vi "InfoGui.vi"(7 "_onebutton(F)":bool caption="one button (F)", 9 "_Arg":variant[](array[variant]), 10 "_Msg":T1) -> (2 "ok":bool)   [LabVIEW 2016]
uses:
  tools/Translator/Translator.Message.ctl
  InfoGui.Action.ctl
  tools/Translator/Translator.FormatMessage.vi
  tools/Translator/Translator.Global.vi
panel:
  out "_loop":i32(ring)=4
  in  "CancelButton":bool
  out "Message":string
  in  "OKButton":bool
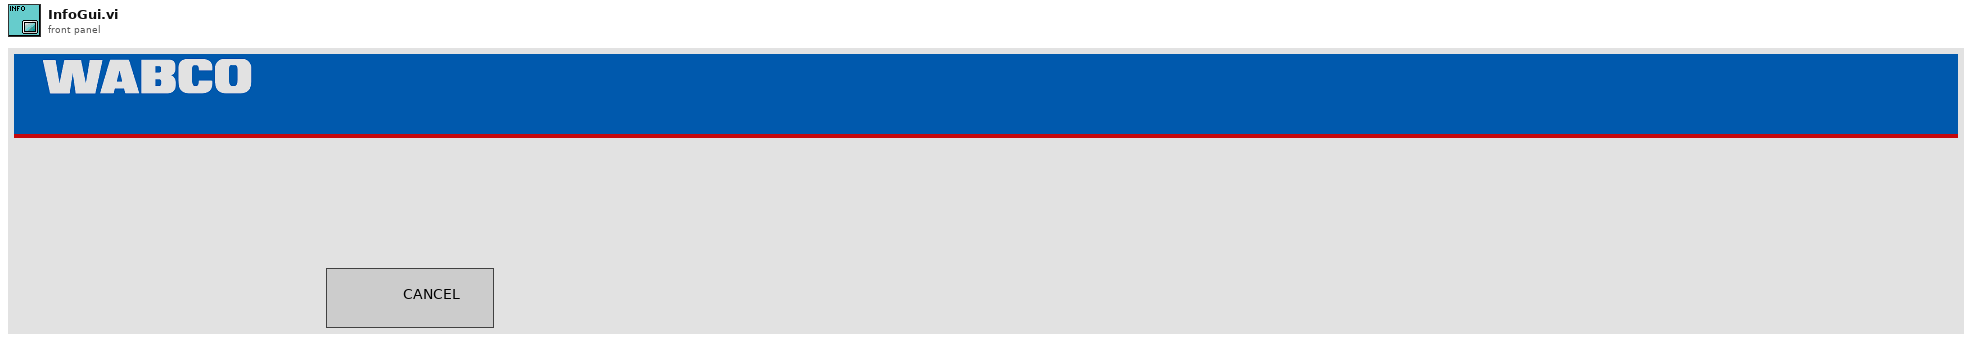
[diagram p1: front panel]
types:
  T1 = typedef "Translator.Message.ctl" = enum16{"-", "Event confirmed", "Log out", "Log in", "Shutdown", "Cancel", "Start", "Begin time", "End time", "Duration", "Service Mode", "Ignore Results", "Serial Format", "On", "Off", "OK", "NOK", "NOK %s", "Home", "Work", "Close", "Open", "In progress...", "Missing", "Empty", "Hardware failure", "Initial", "Default", "Total", "Out of range", "Free disk space is below 1GB - contact technician", "Error %d >> %s", "Error %d >> %s >> %s", "Msg %d >> %s", "Laser msg %d %s", "Laser cmd error %s %d", "Laser cmd failed %s", "Laser cmd warning %s", "Laser disconnected", "Laser status %s", "Laser already started", "Laser job unkonwn %s", "Laser job missing %s", "Laser job select failure %s", "Unable to start laser printing (%s)", "Unable to stop laser printing (%s)", "Laser marking aborted", "Laser marking timeout", "Unable to reset Laser Interlock (%s)", "Unable to trigger Laser. Laser not ready (%s)", "Laser job '%s' coordinates not configured", "Starting %s", "Quitting %s", "Configured", "Initializing", "Quitting", "Loading", "Loaded %d results", "Loaded %d events", "Running", "Stopped", "Summary", "Laser", "Do you want to continue?", "Do you want to delete the configuration?", "The configuration is being used by an order. Unable to delete!", "Press confirm button", "Station is not based. Do you want to exit?", "Station requires changeover. Do you want to run the test?", "Test options are not set as default. Do you want to continue?", "Formatting of WabcoNo is disabled. Do you want to continue?", "Product not detected. Do you want to continue?", "Product scan failed. Do you want to continue?", "Calibration", "Log out?", "System", "All", "IDLE", "Translating...%s", "Not found", "Alarm %s", "Run", "Skip", "Abort", "Repeat", "Please wait...", "Database disconnected", "Database disconnected - changeover disabled!", "Login to database successful", "Login to database failed: %d; %s", "Unable to check the product status of reference %d - database disconnected", "Unable to set the product status of reference %d - database disconnected", "Variant file backup %s", "Read variant (%s)", "Result", "Station armed!", "Station requires changeover!", "Select reference number...", "EMERGENCY BUTTON - press Control button", "EMERGENCY DOOR - press Control button", "Resetting Emergency...", "Unable to reset safety circuit - Emergency Button pressed", "Unable to reset safety circuit - Emergency Side Door open", "Station not based", "Station based", "Station not empty", "Station basing...", "No order", "Press Start to begin new order", "Scanning new order", "Order NOK. Correct or scan again", "Order OK. Press Accept", "Order ready", "Revolver incorrect", "Fork incorrect", "Revolver missing", "Revolver empty", "Container missing", "Offline results", "Offline statistics", "Updating statistics %.1f %%", "DMC Configurator", "Door open", "Close the front door", "Press start button", "Done. Open the front door", "Running...", "Running...%.1f %%", "Pause %s", "Pause %s. NOK container missing", "Pause %s. OK container missing", "Pause %s. Revolver empty", "Pause %s. Revolver missing", "Pause %s. Revolver incorrect", "Pause %s. Fork missing", "Pause %s. Fork incorrect", "Pause %s. Too many failures", "Pause %s. Unloading failure", "Pause %s. One slot is not working", "Pause %s. Part order is done. Empty OK container", "Pause %s. Unable to move product to slot", "Pause %s. Unable to move back product pusher", "Pause %s. Unable to lift product", "Pause %s. Unable to move back product lifter", "Pause %s. Unable to move product arm to Work", "Pause %s. Unable to move product arm to NOK", "Pause %s. Unable to move product arm to OK", "Pause %s. Unable to unsuck the NOK product", "Pause %s. Unable to drop the NOK product", "Pause %s. Product OK missing", "Pause %s. Unable to unsuck the OK product", "Pause %s. Unable to drop the OK product", "Stopping...", "File '%s' is missing", "File '%s' is broken", "File '%s' is running", "Log file started (%s)", "Log file ended (%s)", "Log file stopped (%s)", "Log file ignored (%s)", "Log file exported (%s)", "Log file export failed (%s)", "Wrong serial number in log file", "Wrong reference number in log file", "Test steps are missing", "%s = %.3f", "Process param '%s' not found in DB", "Process param '%s' wrong order", "Process param '%s' value %.3f out of limits (%.3f; %.3f)", "Step%d param '%s' not found in DB", "Step%d param '%s' wrong order", "Step%d param '%s' value %.3f out of limits (%.3f; %.3f)", "Step%d EV '%s' not found in DB", "Step%d EV '%s' wrong order", "\"%s\" not found in DB", "\"%s\" wrong order", "\"%s\" value %.3f out of limits (%.3f; %.3f)", "\"%s\" not found in software", "Process init (%s)", "Process started", "Process restarted", "Process run", "Process done", "Process done - remove OK container", "Process aborted", "Process aborted at work", "Process aborted at home", "Process error", "Process error at home", "Process error at work", "Process close", "Process pause", "Process continue", "Process door open", "Process door close", "Process pause at slot %s due to %s", "Select plate from the order to process", "Do you want to start the process?", "Do you want to continue the process?", "There is unfinished order. Do you want to put the new order?", "Product %s %d OK", "Product %s %d NOK", "Unable to unload the slot %s. Product missing in the slot", "Unable to unload the slot %s. Product already in the arm", "Unable to accept the product as OK. Product missing in slot %s", "Unable to accept the product as OK. Product could not drop into the container at slot %s", "Unable to accept the product as NOK. Product could not drop into the container at slot %s", "Scan failed. Error %s", "Scan failed. Scanner disconnected", "Scan failed. Wrong Wabco number %d, limit (%d,%d)", "Scan failed. Wrong serial number %d, limit (%d,%d)", "Scan failed. Wrong date %d, limit (%d,%d)", "Scan failed. Wrong product wabco number %d (expected %d)", "Scan failed. Wrong product serial number %d (expected > 0)", "Scan OK %s", "Scan failed. Unable to determine table position (%s)", "Scan failed. Timeout", "Tune failed. Scanner disconnected", "Tune failed. Timeout", "%s = %d", "%s = %d->%d", "Unable to set %s = %.2f - Air Pressure Inside off", "Unable to set digital output '%s' = %d", "Unable to activate air pressure inside - timeout", "Unable to activate air pressure inside - aborted", "Unable to switch on Air Main Valve - Air Pressure Inlet off", "Unable to switch on Air Main Valve - Door open", "Unable to switch off Air Main Valve - timeout", "Unable to switch off Air Main Valve - aborted", "Unable to rotate Table - timeout", "Unable to rotate Table - aborted", "Unable to rotate Table - Product Move not in Home position", "Unable to rotate Table - Air Pressure Inside off", "Unable to rotate Table - Product Lift A not in Home position", "Unable to rotate Table - Product Lift B not in Home position", "Unable to rotate Table - unlock before movement timeout", "Unable to rotate Table - lock after movement timeout", "Unable to move Table Lock to %s position - timeout", "Unable to move Table Lock to %s position - aborted", "Unable to move Table Lock to %s position - Air Pressure Inside off", "Unable to move Table Lock to %s position - Table not in position", "Unable to move Product Lift A to %s position - timeout", "Unable to move Product Lift B to %s position - timeout", "Unable to move Product Lift A to %s position - aborted", "Unable to move Product Lift B to %s position - aborted", "Unable to move Product Lift A to %s position - Air Pressure Inside off", "Unable to move Product Lift B to %s position - Air Pressure Inside off", "Unable to move Product Lift A to %s position - Table not locked", "Unable to move Product Lift B to %s position - Table not locked", "Unable to move Product Lift A to %s position - Product Arm not in Work position", "Unable to move Product Lift B to %s position - Product Arm not in Work position", "Unable to set Product Suction Gripper %s to %s - timeout", "Unable to set Product Suction Gripper %s to %s - aborted", "Unable to set Product Suction Gripper %s to %s - Air Pressure Inside off", "Unable to set Product Suction Gripper %s to %s - Table slot unkown", "Unable to move Product Arm to %s position - timeout", "Unable to move Product Arm to %s position - aborted", "Unable to move Product Arm to %s position - Air Pressure Inside off", "Unable to move Product Arm to %s position - Product Lift A not in Home position", "Unable to move Product Arm to %s position - Product Lift B not in Home position", "Unable to move Product to %s position - timeout", "Unable to move Product to %s position - aborted", "Unable to move Product to %s position - Air Pressure Inside off", "Unable to move Product to %s position - Table not in position"}
  T2 = typedef "InfoGui.Action.ctl" = enum32{"idle", "constructor", "destructor", "--- InfoGUI ---"}
  T3 = enum32{"Invalid", "Default", "Floating", "Floating/Auto-Hide", "Modal"}
  T4 = typedef "FestoCPX.Station.ButtonsState.ctl" = cluster{"Start":bool, "Stop":bool, "Control":bool}
  T5 = typedef "LVPositionTypeDef.ctl" = cluster{"Left":i32, "Top":i32}
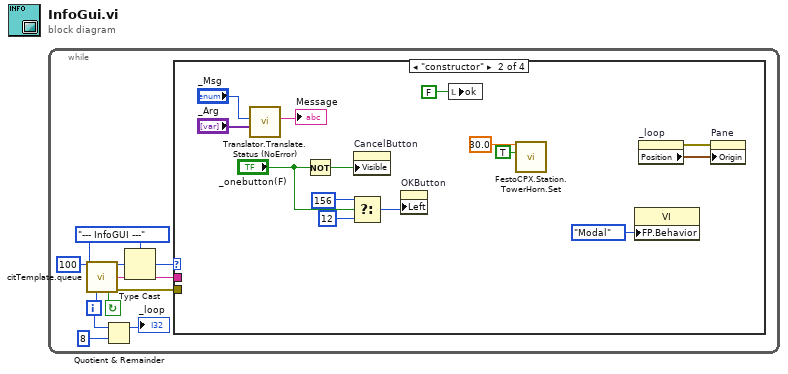
[diagram p0: block diagram]
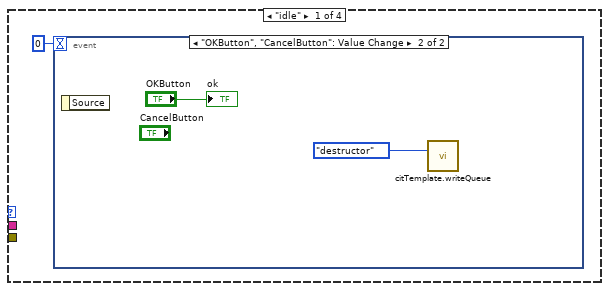
[diagram p2: hidden frame]
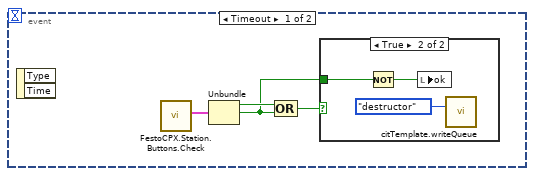
[diagram p3: hidden frame]
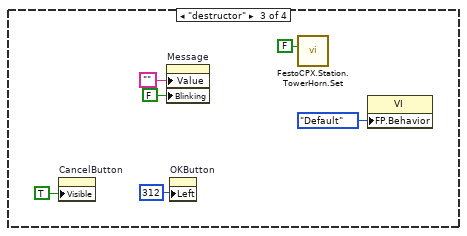
[diagram p5: hidden frame]
diagram:
  n1 = while {
    i -> [w1]
    stop <- w10 continue-if-true
    w4 = InfoGui.Action."--- InfoGUI ---" ("Action")
    n2 = call "citTemplate.queue.vi"("ms timeout (250 ms)"=100, "event enum"=w4, "iteration (-1)"=w1) -> ("event out"=w8:u32, "(flatten) data out"=w5:string, "continue"=w10:bool, "error out"=w6:errorcluster)  [unwired: 2 in, 7 out]
    n3 = Quotient & Remainder(x=w1, y=8) -> (x-y*floor(x/y)=→"_loop":i32)  [unwired: 1 out]
    n4 = Type Cast(type=w4, x=w8) -> (*(type *) &x=w7:T2)
    n5 = case shown="\"constructor\"" w7 {
      tunnel: w6 -> [_ _ _ _]
      tunnel: w5 -> [_ _ _ _]
      frame "idle" {
        n6 = event shown="[1] \"OKButton\", \"CancelButton\": Value Change" {
          selector: _ -> [_ _]
          dyn-events: _ -> [_ _]
          timeout: 0 -> [_ _]
          event Timeout {
            n7 = event-data() -> ()  [unwired: 3 out]
            n8 = call "FestoCPX.Station.Buttons.Check.vi"() -> ("Buttons.State"=w15:T4)  [unwired: 10 in, 1 out]
            n9 = Unbundle(w15) -> ("Start"=w14:bool, "Stop"=w12:bool)  [unwired: 1 out]
            n10 = Compound Arithmetic op=OR(w14, w12) -> (w13:bool)
            n11 = case shown="True" w13 {
              tunnel: w12 -> [_ w17]
              frame False {
              }
              frame True {
                n12 = Not(x=w17) -> (.not. x?=w16:bool)
                n13 = local write "ok"(w16) -> ()
                n14 = call "citTemplate.writeQueue.vi"("event in (if not connected:all statemachine with data event)"=InfoGui.Action."destructor" ("Action")) -> ()  [unwired: 14 in, 1 out]
              }
            }
          }
          event "OKButton", "CancelButton": Value Change {
            n15 = event-data() -> ()  [unwired: 2 out]
            n16 = call "citTemplate.writeQueue.vi"("event in (if not connected:all statemachine with data event)"=InfoGui.Action."destructor" ("Action")) -> ()  [unwired: 14 in, 1 out]
            "ok" <- "OKButton"
          }
        }
      }
      frame "constructor" {
        n17 = call "Translator.Translate.Status (NoError).vi"("Arguments"="_Arg", "msg"="_Msg") -> ("Translated Msg"=→"Message":string)  [unwired: 9 in]
        n18 = Not(x="_onebutton(F)") -> (.not. x?=w33:bool)
        n19 = Select(t=156 ("Position:Left"), s="_onebutton(F)", f=12) -> (s? t:f=w24:i32)
        n20 = property on="CancelButton" class="Bool"("Visible"=w33) -> ()  [unwired: 2 in, 2 out]
        n21 = property on="OKButton" class="Bool"("Left"=w24) -> ()  [unwired: 2 in, 2 out]
        n22 = local write "ok"(FALSE ("_b_ok")) -> ()
        n23 = call "FestoCPX.Station.TowerHorn.Set.vi"("Horn (F)"=TRUE ("Horn1 (F)"), "Period [s] (0)"=30.0) -> ()  [unwired: 9 in, 1 out]
        n24 = property class="VI"("FP.Behavior"=T3."Modal" ("Front Panel Window:Behavior")) -> ()  [unwired: 2 in, 2 out]
        n25 = property on="_loop" class="Ring (strict)"() -> (error out=w25:errorcluster, "Position"=w26:T5)  [unwired: 2 in, 1 out]
        n26 = property on="Pane" class="Pane"(error in=w25, "Origin"=w26) -> ()  [unwired: 1 in, 2 out]
      }
      frame "destructor" {
        n27 = property on="CancelButton" class="Bool"("Visible"=TRUE) -> ()  [unwired: 2 in, 2 out]
        n28 = property on="Message" class="Str"("Value"="", "Blinking"=FALSE) -> ()  [unwired: 2 in, 2 out]
        n29 = property on="OKButton" class="Bool"("Left"=312 ("f")) -> ()  [unwired: 2 in, 2 out]
        n30 = call "FestoCPX.Station.TowerHorn.Set.vi"("Horn (F)"=FALSE ("Horn1 (F)")) -> ()  [unwired: 10 in, 1 out]
        n31 = property class="VI"("FP.Behavior"=T3."Default" ("Front Panel Window:Behavior")) -> ()  [unwired: 2 in, 2 out]
      }
      frame "--- InfoGUI ---" {
      }
    }
  }
